vi "evaluate_operations.vi"(7 "last_status":string, 10 "operation_statuses":string[](array[string]), 11 "stations":string[](array[string])) -> (3 "NOK_stations":string[](array[string]))   [LabVIEW 2019]
uses:
  _misc/AULocalize/SubVIs/Get Localized Phrase Compact Interface 1D.vi
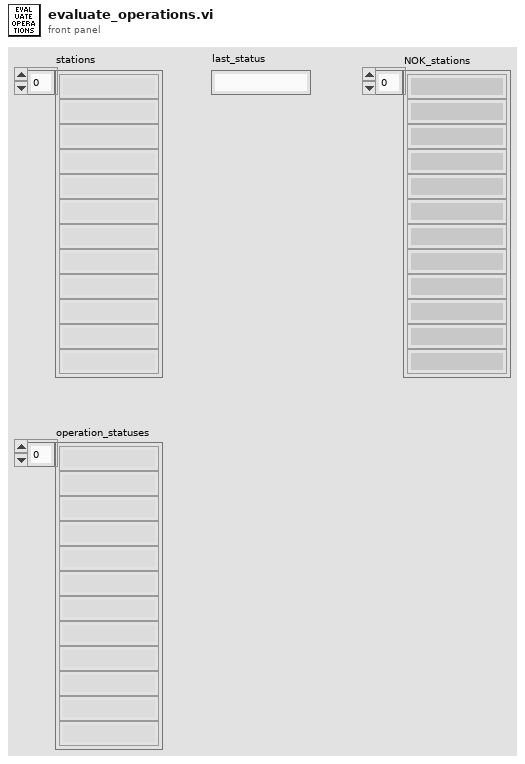
[diagram p1: front panel]
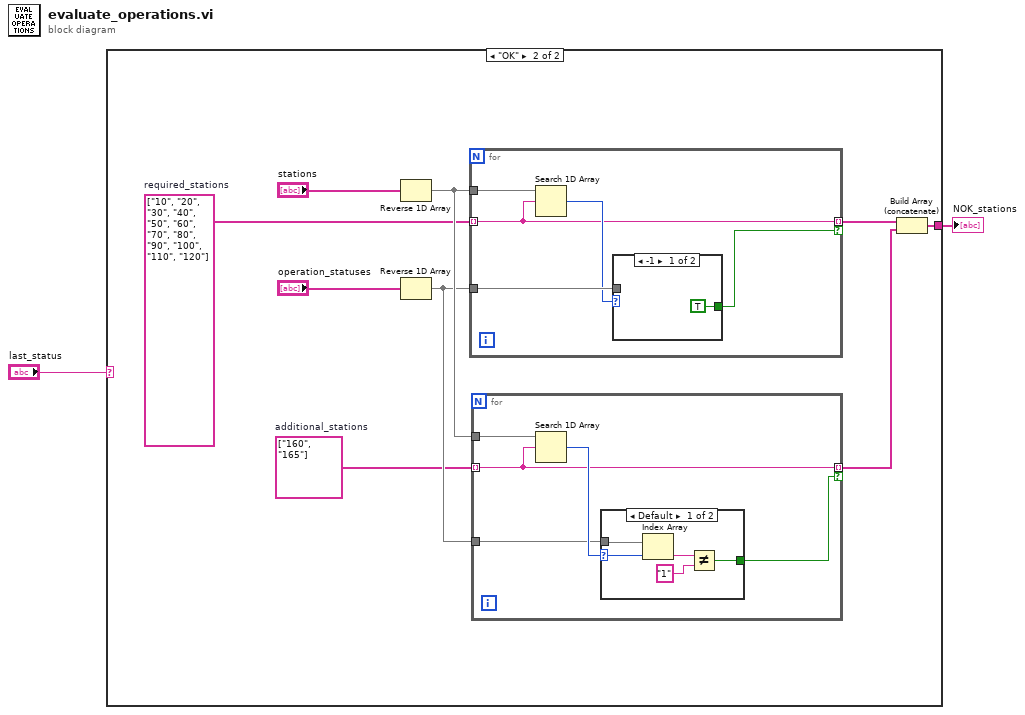
[diagram p0: block diagram]
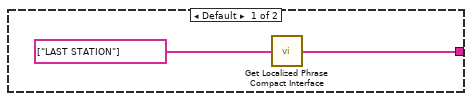
[diagram p2: hidden frame]
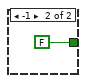
[diagram p3: hidden frame]
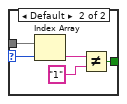
[diagram p4: hidden frame]
diagram:
  n1 = case shown="\"OK\"" "last_status" {
    tunnel: [w3 w5] -> w2
    frame Default {
      n2 = call-poly "Get Localized Phrase Compact Interface.vi"("Key"=string[] ["LAST STATION"]) -> ("Translated Phrase"=w3:string[])
    }
    frame "OK" {
      w8 = string[] ["160", "165"]  # additional_stations
      w9 = string[] ["10", "20", "30", "40", "50", "60", "70", "80", "90", "100", "110", "120"]  # required_stations
      n3 = Reverse 1D Array(array="stations") -> (reversed array=w11:string[])
      n4 = Reverse 1D Array(array="operation_statuses") -> (reversed array=w10:string[])
      n5 = for {
        tunnel: w9 -> [w26] mode=indexing
        tunnel: w11 -> [w29]
        tunnel: w10 -> [w28]
        tunnel: [w26] -> w7 mode=indexing if=w25
        n6 = Search 1D Array(1D array=w29, element=w26) -> (index of element=w27:i32)  [unwired: 1 in]
        n7 = case shown="-1" w27 {
          selector: w27 -> [_ w34]
          tunnel: w28 -> [_ w35]
          tunnel: [TRUE w31] -> w25
          frame -1 {
          }
          frame Default {
            n8 = Index Array(array=w35, index=w34) -> (element=w33:string)
            n9 = Not Equal?(x=w33, y="1") -> (x != y?=w31:bool)
          }
        }
      }
      n10 = for {
        tunnel: w8 -> [w15] mode=indexing
        tunnel: w11 -> [w18]
        tunnel: w10 -> [w16]
        tunnel: [w15] -> w6 mode=indexing if=w14
        n11 = Search 1D Array(1D array=w18, element=w15) -> (index of element=w17:i32)  [unwired: 1 in]
        n12 = case shown="Default" w17 {
          selector: w17 -> [w21 _]
          tunnel: [w19 FALSE] -> w14
          tunnel: w16 -> [w20 _]
          frame Default {
            n13 = Index Array(array=w20, index=w21) -> (element=w22:string)
            n14 = Not Equal?(x=w22, y="1") -> (x != y?=w19:bool)
          }
          frame -1 {
          }
        }
      }
      n15 = Build Array (concatenate)(w7, w6) -> (w5:string[])
    }
  }
  "NOK_stations" <- w2
